vi "PI Terminal.vi"() -> ()   [LabVIEW 2014, in "PiFOC.lvlib"]
doc: "HELP for Terminal.vi\n\nThe terminal VI is a stand-alone application. It first asks the user to specify the full configuration (number of controlled systems, RS-232, GPIB, TCP-IP or DLL communication, communications parameters), then it establishes a connection with a selected system. This will work for all PI devices which support the PI General Command Set, or at least follow the same syntax rules and support the *IDN? and ERR? commands.\n\nAfter starting the VI, the interface parameters of the systems with which to communicate must be selected. For this reason, \"PITerminal.vi\" calls \"PI Ask for Communication Parameters.vi\". Select here the number of connected PI systems that you want to communicate with. For each system, select the appropriate interface parameters. \n\nC-702: Interface = RS232 or TCP/IP, RS232: Input and output HW handshake must be TRUE. Syntax: GCS 1.0; Term char = LF.\n\nC-843: Interface = DLL, DLL for Device = C-843, DLL Interface = Board, Parameter = Board number (1 for first C-843 board). Syntax: GCS 1.0; Term char = LF.\n\nC-843.PM: Interface = DLL, DLL for Device = C-843.PM, DLL Interface = Board, Parameter = Board number (1 for first C-843 board). Syntax: GCS 1.0; Term char = LF.\n\nC-844: Interface = DLL, DLL for Device = C-844, DLL Interface = RS232 or GPIB, Parameter = empty string, RS232 baud rate = 9600. Syntax: GCS 1.0; Term char = LF.\n\nC-865: Interface = DLL, DLL for Device = C-865, DLL Interface = RS232, Parameter = empty string, RS232 baud rate = set as appropriate. Syntax: GCS 1.0; Term char = LF.\n\nC-866: Interface = DLL, DLL for Device = C-866, DLL Interface = RS232 or USB, RS232: Parameter = empty string, RS232 baud rate = set as appropriate, USB: Parameter = Serial no. of system to connect to, Syntax: GCS 1.0; Term char = LF.\n\nC-867: Single Device: Interface = RS232 or DLL, RS232: Input and output HW handshake must be FALSE. DLL (USB): DLL for Device = C-867, DLL Interface = USB, Parameter = Serial no. of system to connect to. DaisyChain: Interface = DLL, DLL for Device = C-867, DLL Interface = RS232_DC, Parameter = Number of device in chain, Register DC: FALSE. Syntax: GCS 2.0; Term char = LF.\n\nC-880, C-848: Interface = RS232 or GPIB, RS232: Input and output HW handshake must be TRUE. Syntax: GCS 1.0; Term char = LF.\n\nC-880K005: Interface = RS232, Input and output HW handshake must be FALSE. Syntax: GCS 1.0; Term char = LF.\n\nC-884: Interface = RS232, TCP/IP or DLL, RS232: Input and output HW handshake must be FALSE. DLL (USB): DLL for Device = PI_GCS2_DLL, DLL Interface = USB, Parameter = Serial no. of system to connect to. Syntax: GCS 2.0; Term char = LF.\n\nE-516: Interface = RS232 or GPIB, RS232: Input and output HW handshake must be TRUE. Syntax: GCS 1.0; Term char = LF.\n\nE-517: Interface = RS232, GPIB, TCP/IP or DLL, RS232: Input and output HW handshake must be TRUE, DLL (USB): DLL for Device = E-517, DLL Interface = USB, Parameter = Serial no. of system to connect to. Syntax: GCS 2.0; Term char = LF.\n\nE-709: Interface = RS232 or DLL, RS232: Input and output HW handshake must be TRUE. DLL (USB): DLL for Device = E-709, DLL Interface = USB, Parameter = Serial no. of system to connect to. Syntax: GCS 2.0; Term char = LF.\n\nE-710: Interface = DLL, DLL for Device = E-710, DLL Interface = RS232 or GPIB, Parameter = empty string. Syntax: GCS 1.0; Term char = LF.\n\nE-712: Interface = RS232, TCP/IP or DLL, RS232: Input and output HW handshake must be TRUE. DLL: DLL for Device = E-712, DLL Interface = USB, Parameter = Serial no. of system to connect to. Syntax: GCS 2.0; Term char = LF.\n\nE-725: Interface = RS232, TCP/IP or DLL, RS232: Input and output HW handshake must be TRUE. DLL: DLL for Device = E-725, DLL Interface = USB, Parameter = Serial no. of system to connect to. Syntax: GCS 2.0; Term char = LF.\n\nE-753: Interface = RS232 or TCP/IP, RS232: Input and output HW handshake must be TRUE. Syntax: GCS 2.0; Term char = LF.\n\nE-755: Single Device: Interface = RS232, Input and output HW handshake must be TRUE. DaisyChain: Interface = DLL, DLL for Device = E-755, DLL Interface = RS232_DC, Parameter = Number of device in chain (first device: 1). Syntax: GCS 2.0; Term char = LF.\n\nE-761: Interface = DLL, DLL for Device = E-761, DLL Interface = Board, Parameter = Board number (1 for first E-761 board). Syntax: GCS 1.0; Term char = LF.\n\nE-816: Interface = RS232 or DLL, RS232: Input and output HW handshake must be TRUE. DLL (USB): DLL for Device = E-816, DLL Interface = USB, Parameter = Serial no. of system to connect to. Syntax: GCS 1.0; Term char = LF. \n\nE-861: Single Device: Interface = RS232 or DLL, RS232: Input and output HW handshake must be FALSE. DLL (USB): DLL for Device = E-861, DLL Interface = USB, Parameter = Serial no. of system to connect to. DaisyChain: Interface = DLL, DLL for Device = E-861, DLL Interface = RS232_DC, Parameter = Number of device in chain (first device: 1), Register DC: FALSE. Syntax: GCS 2.0; Term char = LF.\n\nE-870: Interface = DLL, DLL (USB): DLL for Device = PI_GCS2_DLL, DLL Interface = USB, Parameter = Serial no. of system to connect to.\n Syntax: GCS 2.0; Term char = LF.\n\nE-871: Single Device: Interface = RS232 or DLL, RS232: Input and output HW handshake must be FALSE. DLL (USB): DLL for Device = PI_GCS2_DLL, DLL Interface = USB, Parameter = Serial no. of system to connect to.\n DaisyChain: Interface = DLL, DLL for Device = PI_GCS2_DLL, DLL Interface = RS232_DC or USB_DC, Parameter = Number of device in chain, Register DC: FALSE. Syntax: GCS 2.0; Term char = LF.\n\nHydra, Pollux: Interface = DLL, DLL (TCP/IP and RS-232): DLL for Device = PI_HydraPollux_GCS2_DLL, DLL Interface = RS232 or TCP/IP, Syntax: GCS 2.0; Term char = LF.\n\nF-206, M-8X0: For GCS syntax version = GCS 1.0 (older firmware or compatibility mode, can be set with CSV.vi), Interface = RS232, GPIB (not available for C-887 controller) or TCP/IP., The error status will not be cleared by this VI. The first ERR? query will report a hidden error with error code 1, which will be cleared during system initialization (INI). RS232: Input and output handshake settings must be FALSE. Syntax: GCS 1.0; Term char = LF.\n For GCS syntax version = GCS 2.0 (C-887 Controller), Interface = RS232 or TCP/IP. RS232: Input and output handshake settings must be FALSE. Syntax: GCS 2.0; Term char = LF.\n\nMercury™: Interface = DLL, DLL for Device = Mercury™, DLL Interface = RS232 (even if using USB), Parameter = empty string, RS232 baud rate = same as set on controller hardware. Syntax: GCS 1.0; Term char = LF.\n\nGCS_Mercury: Single Device: Interface = RS232 or DLL, RS232: Input and output HW handshake must be FALSE. DLL (USB): DLL for Device = PI_GCS2_DLL, DLL Interface = USB, Parameter = Serial no. of system to connect to.\n DaisyChain: Interface = DLL, DLL for Device = PI_GCS2_DLL, DLL Interface = RS232_DC, Parameter = Number of device in chain, Register DC: FALSE. Syntax: GCS 2.0; Term char = LF.\n\nIf the chosen timeout value is greater than 1000 ms, it will automatically be set to 1000 ms for a fluid program operation. \n\nIn the upper window (\"Send\") the user can enter commands which will be transmitted to the chosen device one line at a time when the ENTER key is pressed. \nAll controller responses are displayed in the Receive response window, which can be cleared by pressing the Clear Receive Window button or F2. \n\nThe view style of the Receive window can be changed to Show all characters or Hex View using the menu ring above the Receive window.\n\nExit or F10 will terminate the terminal application. \n\nTo send the last command again, just press the ENTER key again. The next line will then show the following entry: \"(Send: cmd)\" with cmd being the command from the line before, which was resent.\n\nWhen the terminal application has just been started, pressing ENTER without entering a command will send \"*IDN?\" to the chosen system. \n\nNew commands can only be inserted into the last line of the Send window. The user can scroll through the history of the Send window using the scroll bar or the cursor up/down keys, but cannot change the history or resend commands by pressing ENTER unless in the last line. Pressing ENTER will always resend the last command, no matter where the cursor is positioned. Selecting text and using copy and paste (Ctrl+C, Ctrl+V) works for single lines, if only the contents of one single line (the command text) is selected and copied, not the full line (including the LineFeed) or multiple lines.\n\nMany of PI's General Command Set compatible devices support single-byte commands. For example, the user can stop a fast scan of a C-880 or F-206 by sending an ASCII 24 (decimal). To enter this command into the Send window simply type a \"#\" followed by the decimal value of the byte to be sent, e.g. enter \"#24\" and presses ENTER to stop a fast scan. An entry \"(Send: *)\" will be added to the original command with * being the corresponding ASCII character of the single byte sent. \n\nPressing F1 or the Help button will pop up a help window. To return to the terminal application, press Esc. If Send ERR? on Exit? is TRUE, an \"ERR?\" query is sent to the device when Exit is pressed to prevent the controller from keeping an error condition produced during the use of the terminal application."
uses:
  PiFOC.lvlib
  Low Level/Communication.llb/Termination character.ctl
  Low Level/Communication.llb/Available DLLs.ctl
panel:
  out "Help string":string="\nHELP for PI Terminal.vi\nPress Esc to return to the terminal application.\n\nThis terminal application works for all PI devices which support the PI General Command Set or at least follow the syntax rules of this command structure and support the commands *IDN? and ERR?.\n\nIn the upper window (\"Send\") the user can enter commands which will be transmitted to the chosen device one line at a time when the ENTER key is pressed. All controller responses are displayed in the Receive response window, which can be cleared by pressing the Clear Receive Window button or F2. The view style of the Receive window can be changed to Show all characters or Hex View using the menu ring above the Receive window.\n\nExit or F10 will terminate the terminal application. \n\nTo send the last command again, just press the ENTER key again. The next line will then show the following entry: \"(Send: cmd)\" with cmd being the command from the line before, which was resent.\nWhen the terminal application has just been started, pressing ENTER without entering a command will send \"*IDN?\" to the chosen system.\n\nNew commands can only be inserted into the last line of the Send window. The user can scroll through the history of the Send window using the scroll bar or the cursor up/down keys, but cannot change the history or resend commands by pressing ENTER unless in the last line. Pressing ENTER will always resend the last command, no matter where the cursor is positioned. Selecting text and using copy and paste (Ctrl+C, Ctrl+V) works for single lines, if only the contents of one single line (the command text) is selected and copied, not the full line (including the LineFeed) or multiple lines.\n\nMany of PI's General Command Set compatible devices support single-byte commands. For example, the user can stop a fast scan of a C-880 or F-206 by sending an ASCII 24 (decimal). To enter this command into the Send window simply type a \"#\" followed by the decimal value of the byte to be sent, e.g. enter \"#24\" and presses ENTER to stop a fast scan. An entry \"(Send: *)\" will be added to the original command with * being the corresponding ASCII character of the single byte sent. \n\nIf Send ERR? on Exit? is TRUE, a \"ERR?\" query is sent to the device when Exit is pressed to prevent the controller from keeping an error condition produced during the use of the terminal application.\n\nC-702: \tInterface = RS232 or TCP/IP, RS232: Input and output HW handshake \tmust \tbe TRUE. Syntax: GCS 1.0; Term char = LF.\n\nC-843: \tInterface = DLL, DLL for Device = C-843, DLL Interface = Board, \tParameter = Board number (1 for first C-843 board). Syntax: GCS 1.0; \tTerm char = LF.\n\nC-843.PM: \tInterface = DLL, DLL for Device = C-843.PM, DLL Interface = Board, \tParameter = Board number (1 for first C-843 board). Syntax: GCS 1.0; \tTerm char = LF.\n\nC-865: \tInterface = DLL, DLL for Device = C-865, DLL Interface = RS232, \tParameter = empty string, RS232 baud rate = set as appropriate. Syntax: \tGCS 1.0; Term char = LF.\n\nC-866: \tInterface = DLL, DLL for Device = C-866, DLL Interface = RS232 or USB, \tRS232: Parameter = empty string, RS232 baud rate = set as appropriate, \tUSB: Parameter = Serial no. of system to connect to, \n\tSyntax: GCS 1.0; Term char = LF.\n\nC-867: \tSingle Device: Interface = RS232 or DLL, RS232: Input and output HW \thandshake must be FALSE. DLL (USB): DLL for Device = C-867, DLL \tInterface = USB, Parameter = Serial no. of system to connect to.\nDaisyChain: Interface = DLL, DLL for Device = C-867, DLL Interface = \tRS232_DC, Parameter = Number of device in chain, \tRegister DC: \tFALSE. Syntax: GCS 2.0; Term char = LF.\n\nC-880, C-848: \tInterface = RS232 or GPIB, RS232: Input and output HW handshake must \tbe TRUE. Syntax: GCS 1.0; Term char = LF.\n\nC-880K005: \tInterface = RS232, Input and output HW handshake must be FALSE. \tSyntax: GCS 1.0; Term char = LF.\n\nC-884: \tInterface = RS232, TCP/IP or DLL, RS232: Input and output HW handshake must be FALSE. DLL (USB): DLL for Device = PI_GCS2_DLL, DLL Interface = USB, Parameter = Serial no. of system to connect to. Syntax: GCS 2.0; Term char = LF.\n\nE-516: \tInterface = RS232 or GPIB, RS232: Input and output HW handshake must \tbe TRUE. Syntax: GCS 1.0; Term char = LF.\n\nE-517: \tInterface = RS232, GPIB, TCP/IP or DLL, RS232: Input and output HW \thandshake must be TRUE, DLL (USB): DLL for Device = E-517, DLL \tInterface = USB, Parameter = Serial no. of system to connect to. \nSyntax: GCS 2.0; Term char = LF.\n\nE-709: \tInterface = RS232 or DLL, RS232: Input and output HW handshake \tmust be TRUE. DLL (USB): DLL for Device = E-709, DLL Interface = USB, \tParameter = Serial no. of system to connect to. Syntax: GCS 2.0; Term \tchar = LF.\n\nE-710:\tInterface = DLL, DLL for Device = E-710, DLL Interface = RS232 or GPIB, \tParameter = empty string. Syntax: GCS 1.0; Term char = LF.\n\nE-712: \tInterface = RS232, TCP/IP or DLL, RS232: Input and output HW \thandshake must be TRUE. DLL: DLL for Device = E-712, DLL Interface = \tUSB, \tParameter = Serial no. of system to connect to. \n\tSyntax: GCS 2.0; Term char = LF.\n\nE-725: \tInterface = RS232, TCP/IP or DLL, RS232: Input and output HW \thandshake must be TRUE. DLL: DLL for Device = E-725, DLL Interface = \tUSB, \tParameter = Serial no. of system to connect to. \nSyntax: GCS 2.0; Term char = LF.\n\nE-753: \tInterface = RS232 or TCP/IP, RS232: Input and output HW handshake \tmust \tbe TRUE. Syntax: GCS 2.0; Term char = LF.\n\nE-755:\tSingle Device: Interface = RS232, Input and output HW handshake must \tbe TRUE. DaisyChain: Interface = DLL, DLL for Device = E-755, DLL \tInterface = RS232_DC, Parameter = Number of device in chain (first \tdevice: 1). Syntax: GCS 2.0; Term char = LF.\n\nE-761:\tInterface = DLL, DLL for Device = E-761, DLL Interface = Board, \tParameter = Board number (1 for first E-761 board). Syntax: GCS 1.0; \tTerm char = LF.\n\nE-816: \tInterface = RS232 or DLL, RS232: Input and output HW handshake must \tbe TRUE. DLL (USB): DLL for Device = E-816, DLL Interface = USB, \tParameter = Serial no. of system to connect to. Syntax: GCS 1.0; Term \tchar = LF. \n\nE-861: \tSingle Device: Interface = RS232 or DLL, RS232: Input and output HW \thandshake must be FALSE. DLL (USB): DLL for Device = E-861, DLL \tInterface = USB, Parameter = Serial no. of system to connect to.\nDaisyChain: Interface = DLL, DLL for Device = E-861, DLL Interface = \tRS232_DC or USB_DC, Parameter = Number of device in chain (first device: 1), \tRegister DC: FALSE. Syntax: GCS 2.0; Term char = LF.\n\nE-870: \tInterface = DLL, DLL (USB): DLL for Device = PI_GCS2_DLL, DLL \tInterface = USB, Parameter = Serial no. of system to connect to.\n\tSyntax: GCS 2.0; Term char = LF.\n\nE-871: Single Device: Interface = RS232 or DLL, RS232: Input and output HW \thandshake must be FALSE. DLL (USB): DLL for Device = \tPI_GCS2_DLL, DLL Interface = USB, Parameter = Serial no. of system to \tconnect to.\n\tDaisyChain: Interface = DLL, DLL for Device = PI_GCS2_DLL, DLL \tInterface = RS232_DC or USB_DC, Parameter = Number of device in \tchain, Register DC: FALSE. Syntax: GCS 2.0; Term char = LF.\n\nHydra, Pollux: \tInterface = DLL, DLL (TCP/IP and RS-232): DLL for Device = \t\t\t\t\tPI_HydraPollux_GCS2_DLL, DLL Interface = RS232 or TCP/IP, Syntax: \t\t\tGCS 2.0; Term char = LF.\n\nF-206, M-8X0: \tFor GCS syntax version = GCS 1.0 (older firmware or compatibility mode, \tcan be set with CSV.vi), Interface = RS232, GPIB (not available for C-887 \tcontroller) or TCP/IP., The error status will not be cleared by this VI. The \tfirst ERR? query will report a hidden error with error code 1, which will be \tcleared during system initialization (INI). RS232: Input and output \thandshake settings must be FALSE. Syntax: GCS 1.0; Term char = \tLF.\n\tFor GCS syntax version = GCS 2.0 (C-887 Controller), Interface = RS232 \tor TCP/IP. RS232: Input and output handshake settings must be FALSE. \tSyntax: GCS 2.0; Term char = LF.\n\nMercury™: \tInterface = DLL, DLL for Device = Mercury™, DLL Interface = RS232 \t(even if using USB), Parameter = empty string, RS232 baud rate = same \tas set on controller hardware, Syntax: GCS 1.0; Term char = LF.\n\nGCS_Mercury: \tSingle Device: Interface = RS232 or DLL, RS232: Input and output HW \thandshake must be FALSE. DLL (USB): DLL for Device = PI_GCS2_DLL, \tDLL Interface = USB, Parameter = Serial no. of system to connect to. \tDaisyChain: Interface = DLL, DLL for Device = PI_GCS2_DLL, DLL \tInterface = RS232_DC or USB_DaisyChain, Parameter = Number of device in chain, \tRegister DC: \tFALSE. Syntax: GCS 2.0; Term char = LF.\n"
  in  "HowTo":string="Start application and choose interface parameters in next window."
  out "TCP/IP Config. System":T1={"Host address/name"="Z-A521-2.pi.ws", "Port"=3000, "Board"=0, "Timeout"=5000}
  in  "ERR? on exit?":bool=TRUE
  out "error out":T2
  out "GPIB Configuration system":T3={"bus"=0, "address"=4, "mode"=0, "Timeout"=1000}
  in  "Hide help":bool
  in  "Show help":bool
  in  "View style":u16(ring) items=["Normal view", "Show all characters", "Hex View"]
  out "error":bool
  in  "Send":bool
  in  "Clear":bool
  in  "Exit":bool
  out "Receive":string
  in  "System No.":i32=1 min=1 step=1
  out "Interface":u16(ring) items=["RS232", "GPIB", "DLL", "TCP/IP"]
  out "System ind.":i32=1
  out "System":i32=1
  out "RS232 Config. System":T4={"RS232 Portnumber"=0, "Timeout"=1000, "Baudrate"=57600, "Handshake"=0} {"Handshake" items=["None", "HW", "XON/XOFF"]; "RS232 Portnumber" items=["COM1", "COM2", "COM3", "COM4", "COM5", "COM6", "COM7", "COM8", "COM9", "COM10", "COM11", "COM12", "COM13", "COM14", "COM15", "COM16", "COM17", "COM18", "COM19", "COM20", "COM21", "COM22", "COM23", "COM24", "COM25", "COM26", "COM27", "COM28", "COM29", "COM30"]}
  in  "Send":string="*IDN?\n"
  out "Term.char":T5
  out "DLL for Device":T6 items=["C-843", "C-844", "E-710", "C-843.PM", "C-865", "E-761", "Mercury", "E-755", "E-753", "C-866", "E-712", "E-725", "E-861", "C-867", "E-517", "E-816", "E-709", "PI_GCS2_DLL", "HydraPollux"]
  # "Terminal"
  # "If chosen timeout value is > 1000 ms, \nit will be set to 300 ms."
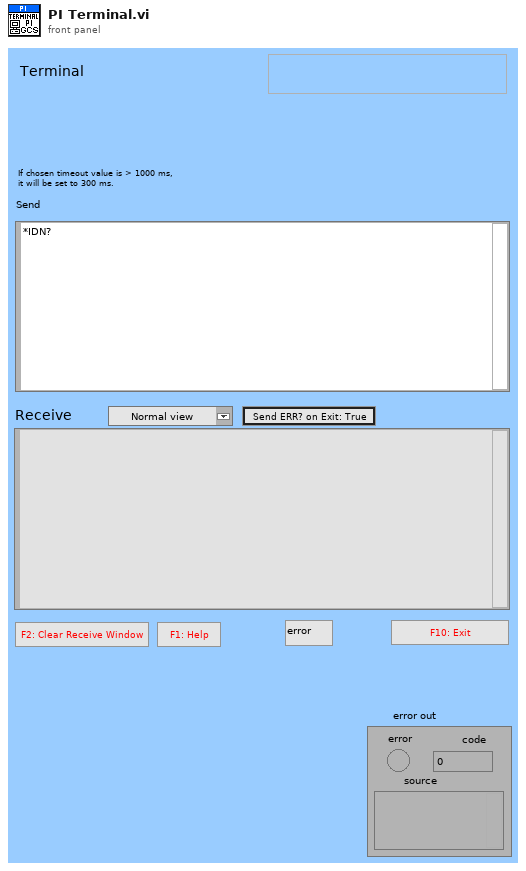
[diagram p1: front panel]
types:
  T1 = cluster{"Host address/name":string, "Port":i32, "Board":i32, "Timeout":i32}
  T2 = cluster{"error":bool, "code":i32, "source":string}
  T3 = cluster{"bus":i16, "address":i16, "mode":i16, "Timeout":i32}
  T4 = cluster{"RS232 Portnumber":i32, "Timeout":i32, "Baudrate":u32, "Handshake":u16}
  T5 = typedef "PiFOC.lvlib/Termination character.ctl" = enum16{"LF", "CR", "LFCR", "CRLF"}
  T6 = typedef "PiFOC.lvlib/Available DLLs.ctl" = u16
  T7 = cluster{"data bits":u16, "stop bits":enum16{"1 bit", "1.5 bits", "2 bits"}, "parity":enum16{"no parity", "odd parity", "even parity", "mark parity", "space parity"}}
  T8 = cluster{"Host address/name":string, "Port":i32, "Board":i32}[]
  T9 = cluster{"input XON/XOFF":bool, "input HW Handshake":bool, "input alt HW HShk":bool, "output XON/XOFF":bool, "output HW Handshake":bool, "output alt HW HShk":bool, "XOFF byte ":u8, "XON byte":u8, "parity error byte":u16}[]
  T10 = typedef "PiFOC.lvlib/Available interfaces.ctl" = u16
  T11 = cluster{"RS232 Portnumber":u16, "Timeout":u32, "RS232 baud rate":u32, "Interface":T10, "GPIB Bus":i16, "GPIB address":i16, "GPIB Mode":i16}[]
  T12 = typedef "PiFOC.lvlib/Available DLL interfaces.ctl" = u16
  T13 = cluster{"DLL for Device":T6, "DLL Interface":T12, "Parameter":string}[]
  T14 = cluster{"RS232 Portnumber":u16, "Timeout":u32, "RS232 baud rate":u32, "Interface":T10, "GPIB Bus":i16, "GPIB address":i16, "GPIB Mode":i16}
  T15 = cluster{"Portnumber":u32, "Timeout":i32, "Baudrate":u32, "Handshake":u16}
  T16 = cluster{"data bits":u16, "stop bits":enum16{"1 bit", "1.5 bits", "2 bits"}, "parity":enum16{"no parity", "odd parity", "even parity", "mark parity", "space parity"}}[]
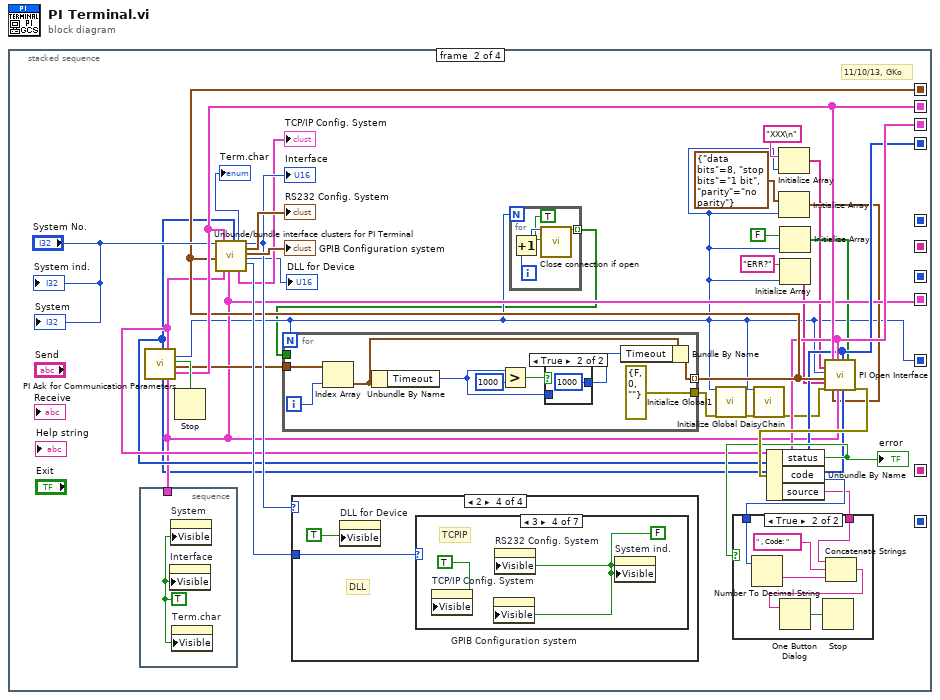
[diagram p0: block diagram]
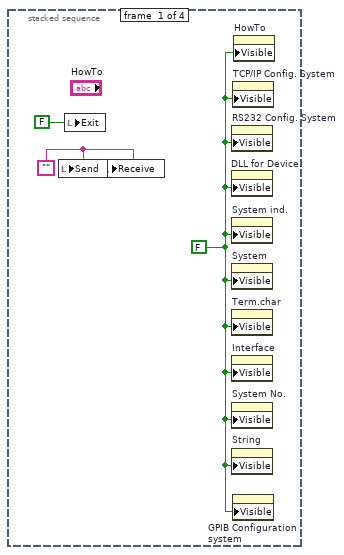
[diagram p2: hidden frame]
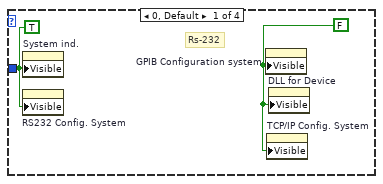
[diagram p3: hidden frame]
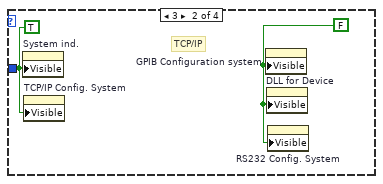
[diagram p4: hidden frame]
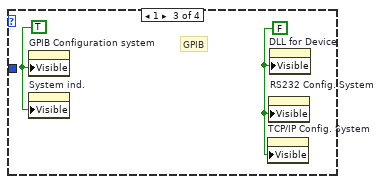
[diagram p5: hidden frame]
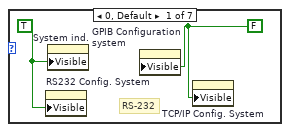
[diagram p6: hidden frame]
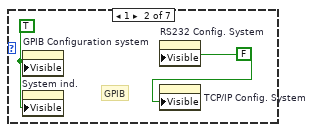
[diagram p7: hidden frame]
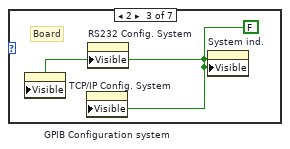
[diagram p8: hidden frame]
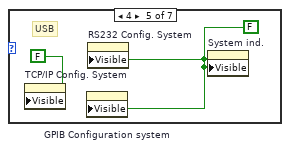
[diagram p9: hidden frame]
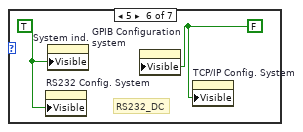
[diagram p10: hidden frame]
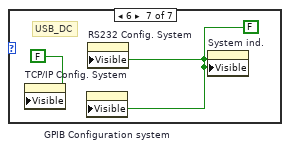
[diagram p11: hidden frame]
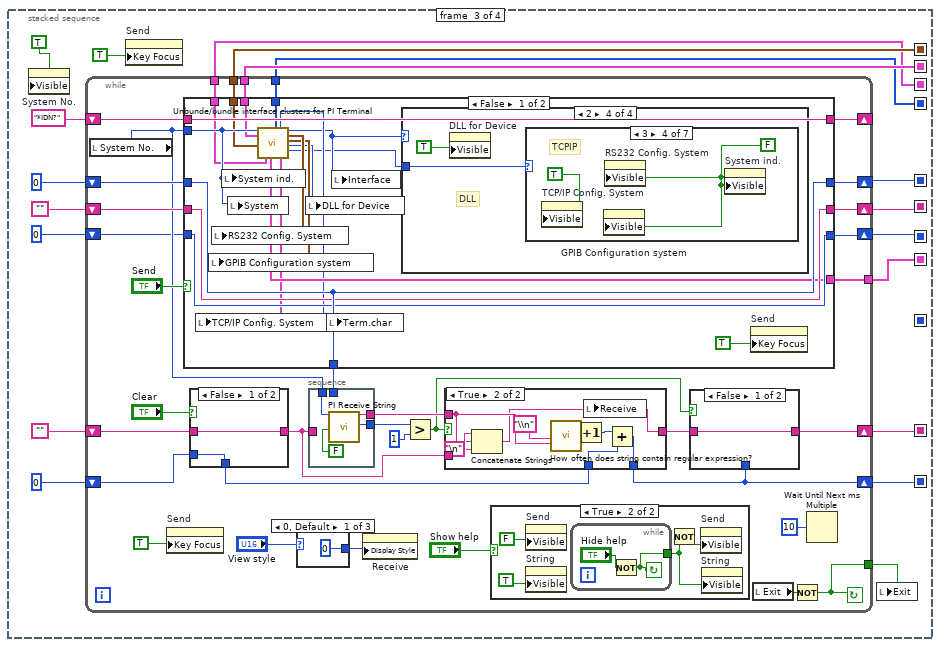
[diagram p14: hidden frame]
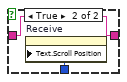
[diagram p16: hidden frame]
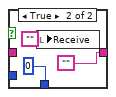
[diagram p17: hidden frame]
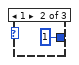
[diagram p19: hidden frame]
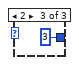
[diagram p20: hidden frame]
diagram:
  n1 = stacked-sequence {
    seq-local: [_ w24 _ _] -> [_ _ w97 _]
    seq-local: [_ w32 _ _] -> [_ _ w96 _]
    seq-local: [_ w19 _ _] -> [_ _ w87 _]
    seq-local: [_ _ w86 _] -> [_ _ _ w246]
    seq-local: [_ _ w85 _] -> [_ _ _ w245]
    seq-local: [_ _ w84 _] -> [_ _ _ w247]
    seq-local: [_ _ w83 _] -> [_ _ _ w248]
    seq-local: [_ _ w82 _] -> [_ _ _ w249]
    seq-local: [_ w21 _ _] -> [_ _ w81 _]
    seq-local: [_ w20 _ _] -> [_ _ w80 _]
    seq-local: [_ w7 _ _] -> [_ _ _ w243]
    frame #0 {
      w1 = FALSE ("Visible")
      w3 = ""
      n2 = local write "Send"(w3) -> ()
      n3 = local write "Exit"(FALSE ("error")) -> ()
      n4 = local write "Receive"(w3) -> ()
      n5 = property on="RS232 Config. System" class="Clust (strict)"("Visible"=w1) -> ()  [unwired: 2 in, 2 out]
      n6 = property on="DLL for Device" class="Ring (strict)"("Visible"=w1) -> ()  [unwired: 2 in, 2 out]
      n7 = property on="System ind." class="DigNum (strict)"("Visible"=w1) -> ()  [unwired: 2 in, 2 out]
      n8 = property on="System" class="DigNum (strict)"("Visible"=w1) -> ()  [unwired: 2 in, 2 out]
      n9 = property on="Term.char" class="Enum (strict)"("Visible"=w1) -> ()  [unwired: 2 in, 2 out]
      n10 = property on="Interface" class="Ring (strict)"("Visible"=w1) -> ()  [unwired: 2 in, 2 out]
      n11 = property on="System No." class="DigNum (strict)"("Visible"=w1) -> ()  [unwired: 2 in, 2 out]
      n12 = property on="String" class="Str"("Visible"=w1) -> ()  [unwired: 2 in, 2 out]
      n13 = property on="TCP/IP Config. System" class="Clust (strict)"("Visible"=w1) -> ()  [unwired: 2 in, 2 out]
      n14 = property on="GPIB Configuration system" class="Clust (strict)"("Visible"=w1) -> ()  [unwired: 2 in, 2 out]
      n15 = property on="HowTo" class="Str"("Visible"=w1) -> ()  [unwired: 2 in, 2 out]
    }
    frame #1 {
      # "11/10/13, GKo"
      n16 = call "PI Ask for Communication Parameters.vi"() -> ("Termination character out"=w20:T5[], "Syntax out"=w18:enum16{"GCS 1.0", "GCS 2.0"}[], "TCP/IP Configuration out"=w21:T8, "Flow control out"=w19:T9, "How many\nsystems? out"=w7:i32, "Abort out"=w35:bool, "Interface configuration out"=w25:T11, "DLL Interface\nconfiguration out"=w32:T13)  [unwired: 12 out]
      n17 = stacked-sequence {
        tunnel: w19 -> [_]
        frame #0 {
          w41 = TRUE ("Visible")
          n18 = property on="Interface" class="Ring (strict)"("Visible"=w41) -> ()  [unwired: 2 in, 2 out]
          n19 = property on="System" class="DigNum (strict)"("Visible"=w41) -> ()  [unwired: 2 in, 2 out]
          n20 = property on="Term.char" class="Enum (strict)"("Visible"=w41) -> ()  [unwired: 2 in, 2 out]
        }
      }
      n21 = Stop(stop? (T)=w35) -> ()
      n22 = for {
        N: w7 -> [_]
        tunnel: [w37] -> w6 mode=indexing
        i -> [w40]
        n23 = Increment(x=w40) -> (x+1=w39:i32)
        n24 = call "Close connection if open.vi"("System no."=w39, "Close DaisyChain"=TRUE) -> ("Was connected?"=w37:bool)  [unwired: 1 in, 16 out]
      }
      n25 = for {
        N: w7 -> [_]
        tunnel: w25 -> [w76]
        tunnel: [w75] -> w24 mode=indexing
        tunnel: w6 -> [_]
        tunnel: [errorcluster {"status"=FALSE, "code"=0, "source"=""} ("error in")] -> w5
        i -> [w77]
        n26 = Index Array(array=w76, index=w77) -> (element=w72:T14)
        n27 = Unbundle By Name(w72) -> ("Timeout"=w71:u32)
        n28 = Greater?(x=w71, y=u32 1000) -> (0:w70:bool)
        n29 = case shown="True" w70 {
          tunnel: [w78 1000] -> w73
          tunnel: w71 -> [w78 _]
          frame False {
          }
          frame True {
          }
        }
        n30 = Bundle By Name(cluster=w72, "Timeout"=w73) -> (w75:T14)
      }
      n31 = call "Unbunde/bundle interface clusters for PI Terminal.vi"("System No."="System No.", "Interface configuration"=w24, "DLL Interface\nconfiguration"=w32, "TCP/IP Configuration"=w21, "Flow control"=w19, "Termination character"=w20) -> ("Term.char"=→"Term.char":T5, "TCP/IP Config. System"=→"TCP/IP Config. System":T1, "Interface"=w28:T10, "RS232 configuration system"=→"RS232 Config. System":T15, "GPIB configuration system"=→"GPIB Configuration system":T3, "DLL for Device"=→"DLL for Device":T6, "DLL interface"=w27:T12)  [unwired: 7 out]
      "Interface" <- w28
      n32 = case shown="2" w28 {
        tunnel: w27 -> [_ _ _ w49]
        frame 0, Default {
          w42 = FALSE ("Write Attribute")
          w43 = TRUE ("Write Attribute")
          # "Rs-232"
          n33 = property on="System ind." class="DigNum (strict)"("Visible"=w43) -> ()  [unwired: 2 in, 2 out]
          n34 = property on="RS232 Config. System" class="Clust (strict)"("Visible"=w43) -> ()  [unwired: 2 in, 2 out]
          n35 = property on="GPIB Configuration system" class="Clust (strict)"("Visible"=w42) -> ()  [unwired: 2 in, 2 out]
          n36 = property on="TCP/IP Config. System" class="Clust (strict)"("Visible"=w42) -> ()  [unwired: 2 in, 2 out]
          n37 = property on="DLL for Device" class="Ring (strict)"("Visible"=w42) -> ()  [unwired: 2 in, 2 out]
        }
        frame 3 {
          w44 = FALSE ("Write Attribute")
          w45 = TRUE ("Write Attribute")
          # "TCP/IP"
          n38 = property on="System ind." class="DigNum (strict)"("Visible"=w45) -> ()  [unwired: 2 in, 2 out]
          n39 = property on="TCP/IP Config. System" class="Clust (strict)"("Visible"=w45) -> ()  [unwired: 2 in, 2 out]
          n40 = property on="GPIB Configuration system" class="Clust (strict)"("Visible"=w44) -> ()  [unwired: 2 in, 2 out]
          n41 = property on="DLL for Device" class="Ring (strict)"("Visible"=w44) -> ()  [unwired: 2 in, 2 out]
          n42 = property on="RS232 Config. System" class="Clust (strict)"("Visible"=w44) -> ()  [unwired: 2 in, 2 out]
        }
        frame 1 {
          w47 = TRUE ("Write Attribute")
          w46 = FALSE ("Write Attribute")
          # "GPIB"
          n43 = property on="GPIB Configuration system" class="Clust (strict)"("Visible"=w47) -> ()  [unwired: 2 in, 2 out]
          n44 = property on="System ind." class="DigNum (strict)"("Visible"=w47) -> ()  [unwired: 2 in, 2 out]
          n45 = property on="TCP/IP Config. System" class="Clust (strict)"("Visible"=w46) -> ()  [unwired: 2 in, 2 out]
          n46 = property on="RS232 Config. System" class="Clust (strict)"("Visible"=w46) -> ()  [unwired: 2 in, 2 out]
          n47 = property on="DLL for Device" class="Ring (strict)"("Visible"=w46) -> ()  [unwired: 2 in, 2 out]
        }
        frame 2 {
          # "DLL"
          n48 = property on="DLL for Device" class="Ring (strict)"("Visible"=TRUE ("Write Attribute")) -> ()  [unwired: 2 in, 2 out]
          n49 = case shown="3" w49 {
            frame 0, Default {
              w50 = FALSE ("Write Attribute")
              w51 = TRUE ("Write Attribute")
              # "RS-232"
              n50 = property on="RS232 Config. System" class="Clust (strict)"("Visible"=w51) -> ()  [unwired: 2 in, 2 out]
              n51 = property on="System ind." class="DigNum (strict)"("Visible"=w51) -> ()  [unwired: 2 in, 2 out]
              n52 = property on="GPIB Configuration system" class="Clust (strict)"("Visible"=w50) -> ()  [unwired: 2 in, 2 out]
              n53 = property on="TCP/IP Config. System" class="Clust (strict)"("Visible"=w50) -> ()  [unwired: 2 in, 2 out]
            }
            frame 1 {
              w53 = TRUE ("Write Attribute")
              w52 = FALSE ("Write Attribute")
              # "GPIB"
              n54 = property on="GPIB Configuration system" class="Clust (strict)"("Visible"=w53) -> ()  [unwired: 2 in, 2 out]
              n55 = property on="System ind." class="DigNum (strict)"("Visible"=w53) -> ()  [unwired: 2 in, 2 out]
              n56 = property on="RS232 Config. System" class="Clust (strict)"("Visible"=w52) -> ()  [unwired: 2 in, 2 out]
              n57 = property on="TCP/IP Config. System" class="Clust (strict)"("Visible"=w52) -> ()  [unwired: 2 in, 2 out]
            }
            frame 2 {
              w54 = FALSE ("Write Attribute")
              # "Board"
              n58 = property on="TCP/IP Config. System" class="Clust (strict)"("Visible"=w54) -> ()  [unwired: 2 in, 2 out]
              n59 = property on="GPIB Configuration system" class="Clust (strict)"("Visible"=w54) -> ()  [unwired: 2 in, 2 out]
              n60 = property on="RS232 Config. System" class="Clust (strict)"("Visible"=w54) -> ()  [unwired: 2 in, 2 out]
              n61 = property on="System ind." class="DigNum (strict)"("Visible"=w54) -> ()  [unwired: 2 in, 2 out]
            }
            frame 3 {
              w56 = FALSE ("Write Attribute")
              # "TCPIP"
              n62 = property on="TCP/IP Config. System" class="Clust (strict)"("Visible"=TRUE) -> ()  [unwired: 2 in, 2 out]
              n63 = property on="GPIB Configuration system" class="Clust (strict)"("Visible"=w56) -> ()  [unwired: 2 in, 2 out]
              n64 = property on="RS232 Config. System" class="Clust (strict)"("Visible"=w56) -> ()  [unwired: 2 in, 2 out]
              n65 = property on="System ind." class="DigNum (strict)"("Visible"=w56) -> ()  [unwired: 2 in, 2 out]
            }
            frame 4 {
              w58 = FALSE ("Write Attribute")
              # "USB"
              n66 = property on="TCP/IP Config. System" class="Clust (strict)"("Visible"=FALSE) -> ()  [unwired: 2 in, 2 out]
              n67 = property on="GPIB Configuration system" class="Clust (strict)"("Visible"=w58) -> ()  [unwired: 2 in, 2 out]
              n68 = property on="RS232 Config. System" class="Clust (strict)"("Visible"=w58) -> ()  [unwired: 2 in, 2 out]
              n69 = property on="System ind." class="DigNum (strict)"("Visible"=w58) -> ()  [unwired: 2 in, 2 out]
            }
            frame 5 {
              w59 = FALSE ("Write Attribute")
              w60 = TRUE ("Write Attribute")
              # "RS232_DC"
              n70 = property on="RS232 Config. System" class="Clust (strict)"("Visible"=w60) -> ()  [unwired: 2 in, 2 out]
              n71 = property on="System ind." class="DigNum (strict)"("Visible"=w60) -> ()  [unwired: 2 in, 2 out]
              n72 = property on="GPIB Configuration system" class="Clust (strict)"("Visible"=w59) -> ()  [unwired: 2 in, 2 out]
              n73 = property on="TCP/IP Config. System" class="Clust (strict)"("Visible"=w59) -> ()  [unwired: 2 in, 2 out]
            }
            frame 6 {
              w62 = FALSE ("Write Attribute")
              # "USB_DC"
              n74 = property on="TCP/IP Config. System" class="Clust (strict)"("Visible"=FALSE) -> ()  [unwired: 2 in, 2 out]
              n75 = property on="GPIB Configuration system" class="Clust (strict)"("Visible"=w62) -> ()  [unwired: 2 in, 2 out]
              n76 = property on="RS232 Config. System" class="Clust (strict)"("Visible"=w62) -> ()  [unwired: 2 in, 2 out]
              n77 = property on="System ind." class="DigNum (strict)"("Visible"=w62) -> ()  [unwired: 2 in, 2 out]
            }
          }
        }
      }
      n78 = call "Initialize Global1.vi"("System no."=w7, "error in"=w5) -> ("error out"=w17:errorcluster)  [unwired: 17 out]
      n79 = call "Initialize Global DaisyChain.vi"("System no."=w7, "error in"=w17) -> ("error out"=w16:errorcluster)  [unwired: 17 out]
      n80 = Initialize Array("XXX\n", w7) -> (w9:string[])
      n81 = Initialize Array(T7 {"data bits"=8, "stop bits"=enum."1 bit", "parity"=enum."no parity"} ("Bit settings and parity"), w7) -> (w11:T16)
      n82 = Initialize Array(FALSE ("Register DC"), w7) -> (w15:bool[])
      n83 = Initialize Array("ERR?", w7) -> (w13:string[])
      n84 = call "PI Open Interface.vi"("Interface clear"=w9, "Number of systems"=w7, "Interface configuration"=w24, "Strings to send"=w13, "error in"=w16, "DLL Interface\nConfiguration"=w32, "Bit settings and parity"=w11, "TCP/IP\nConfiguration"=w21, "Flow control"=w19, "Termination character"=w20, "Syntax"=w18, "Register DC"=w15) -> ("error out"=w36:errorcluster)  [unwired: 7 out]
      n85 = Unbundle By Name(w36) -> ("status"=w26:bool, "code"=w34:i32, "source"=w33:string)
      "error" <- w26
      n86 = case shown="True" w26 {
        tunnel: w34 -> [_ w67]
        tunnel: w33 -> [_ w66]
        frame False {
        }
        frame True {
          n87 = Number To Decimal String(number=w67) -> (decimal integer string=w64:string)  [unwired: 1 out]
          n88 = Concatenate Strings(w66, " , Code: " ("Substring"), w64) -> (w63:string)
          n89 = One Button Dialog(message=w63) -> (true=w68:bool)  [unwired: 1 out]
          n90 = Stop(stop? (T)=w68) -> ()
        }
      }
      "System ind." <- "System No."
      "System" <- "System No."
    }
    frame #2 {
      n91 = property on="System No." class="DigNum (strict)"("Visible"=TRUE ("Write Attribute")) -> ()  [unwired: 2 in, 2 out]
      n92 = while {
        tunnel: w87 -> [w102]
        tunnel: [w103] -> w88
        shift-left: 0 -> [w116]
        shift-right: [w115] -> w84
        shift-left: 0 -> [w112]
        shift-right: [w106] -> w85
        shift-left: "" -> [w113]
        shift-right: [w107] -> w86
        shift-left: "" -> [w124]
        shift-right: [w123] -> w83
        shift-left: 0 -> [w128]
        shift-right: [w127] -> w82
        tunnel: w96 -> [w132]
        tunnel: w97 -> [w133]
        shift-left: "*IDN?" -> [w130]
        shift-right: [w129] -> _
        tunnel: w81 -> [w100]
        tunnel: w80 -> [w99]
        stop <- w103 continue-if-true
        n93 = local read "System No."() -> (w121:i32)
        n94 = property on="Send" class="Str"("Key Focus"=TRUE ("Write Attribute")) -> ()  [unwired: 2 in, 2 out]
        n95 = case shown="False" "Send" {
          tunnel: w121 -> [w178 w224]
          tunnel: w133 -> [w177 _]
          tunnel: w132 -> [w176 _]
          tunnel: w130 -> [w183 w222]
          tunnel: [w183 w219] -> w129
          tunnel: w128 -> [w182 w210]
          tunnel: [w182 w207] -> w127
          tunnel: w124 -> [w179 w218]
          tunnel: [w179 w214] -> w123
          tunnel: [w182 w207] -> w122
          tunnel: w116 -> [w180 w213]
          tunnel: [w180 w209] -> w115
          tunnel: w102 -> [w172 _]
          tunnel: w100 -> [w171 _]
          tunnel: w99 -> [w170 _]
          frame False {
            n96 = local write "System ind."(w178) -> ()
            n97 = local write "System"(w178) -> ()
            n98 = call "Unbunde/bundle interface clusters for PI Terminal.vi"("System No."=w178, "Interface configuration"=w177, "DLL Interface\nconfiguration"=w176, "TCP/IP Configuration"=w171, "Flow control"=w172, "Termination character"=w170) -> ("Term.char"=w168:T5, "TCP/IP Config. System"=w169:T1, "Interface"=w167:T10, "RS232 configuration system"=w175:T15, "GPIB configuration system"=w174:T3, "DLL for Device"=w173:T6, "DLL interface"=w166:T12)  [unwired: 7 out]
            n99 = local write "TCP/IP Config. System"(w169) -> ()
            n100 = local write "GPIB Configuration system"(w174) -> ()
            n101 = local write "RS232 Config. System"(w175) -> ()
            n102 = local write "DLL for Device"(w173) -> ()
            n103 = local write "Term.char"(w168) -> ()
            n104 = local write "Interface"(w167) -> ()
            n105 = case shown="2" w167 {
              tunnel: w166 -> [_ _ _ w191]
              frame 0, Default {
                w184 = FALSE ("Write Attribute")
                w185 = TRUE ("Write Attribute")
                # "Rs-232"
                n106 = property on="System ind." class="DigNum (strict)"("Visible"=w185) -> ()  [unwired: 2 in, 2 out]
                n107 = property on="RS232 Config. System" class="Clust (strict)"("Visible"=w185) -> ()  [unwired: 2 in, 2 out]
                n108 = property on="GPIB Configuration system" class="Clust (strict)"("Visible"=w184) -> ()  [unwired: 2 in, 2 out]
                n109 = property on="TCP/IP Config. System" class="Clust (strict)"("Visible"=w184) -> ()  [unwired: 2 in, 2 out]
                n110 = property on="DLL for Device" class="Ring (strict)"("Visible"=w184) -> ()  [unwired: 2 in, 2 out]
              }
              frame 3 {
                w186 = FALSE ("Write Attribute")
                w187 = TRUE ("Write Attribute")
                # "TCP/IP"
                n111 = property on="System ind." class="DigNum (strict)"("Visible"=w187) -> ()  [unwired: 2 in, 2 out]
                n112 = property on="TCP/IP Config. System" class="Clust (strict)"("Visible"=w187) -> ()  [unwired: 2 in, 2 out]
                n113 = property on="GPIB Configuration system" class="Clust (strict)"("Visible"=w186) -> ()  [unwired: 2 in, 2 out]
                n114 = property on="DLL for Device" class="Ring (strict)"("Visible"=w186) -> ()  [unwired: 2 in, 2 out]
                n115 = property on="RS232 Config. System" class="Clust (strict)"("Visible"=w186) -> ()  [unwired: 2 in, 2 out]
              }
              frame 1 {
                w189 = TRUE ("Write Attribute")
                w188 = FALSE ("Write Attribute")
                # "GPIB"
                n116 = property on="GPIB Configuration system" class="Clust (strict)"("Visible"=w189) -> ()  [unwired: 2 in, 2 out]
                n117 = property on="System ind." class="DigNum (strict)"("Visible"=w189) -> ()  [unwired: 2 in, 2 out]
                n118 = property on="TCP/IP Config. System" class="Clust (strict)"("Visible"=w188) -> ()  [unwired: 2 in, 2 out]
                n119 = property on="RS232 Config. System" class="Clust (strict)"("Visible"=w188) -> ()  [unwired: 2 in, 2 out]
                n120 = property on="DLL for Device" class="Ring (strict)"("Visible"=w188) -> ()  [unwired: 2 in, 2 out]
              }
              frame 2 {
                # "DLL"
                n121 = property on="DLL for Device" class="Ring (strict)"("Visible"=TRUE ("Write Attribute")) -> ()  [unwired: 2 in, 2 out]
                n122 = case shown="3" w191 {
                  frame 0, Default {
                    w192 = FALSE ("Write Attribute")
                    w193 = TRUE ("Write Attribute")
                    # "RS-232"
                    n123 = property on="RS232 Config. System" class="Clust (strict)"("Visible"=w193) -> ()  [unwired: 2 in, 2 out]
                    n124 = property on="System ind." class="DigNum (strict)"("Visible"=w193) -> ()  [unwired: 2 in, 2 out]
                    n125 = property on="GPIB Configuration system" class="Clust (strict)"("Visible"=w192) -> ()  [unwired: 2 in, 2 out]
                    n126 = property on="TCP/IP Config. System" class="Clust (strict)"("Visible"=w192) -> ()  [unwired: 2 in, 2 out]
                  }
                  frame 1 {
                    w195 = TRUE ("Write Attribute")
                    w194 = FALSE ("Write Attribute")
                    # "GPIB"
                    n127 = property on="GPIB Configuration system" class="Clust (strict)"("Visible"=w195) -> ()  [unwired: 2 in, 2 out]
                    n128 = property on="System ind." class="DigNum (strict)"("Visible"=w195) -> ()  [unwired: 2 in, 2 out]
                    n129 = property on="RS232 Config. System" class="Clust (strict)"("Visible"=w194) -> ()  [unwired: 2 in, 2 out]
                    n130 = property on="TCP/IP Config. System" class="Clust (strict)"("Visible"=w194) -> ()  [unwired: 2 in, 2 out]
                  }
                  frame 2 {
                    w196 = FALSE ("Write Attribute")
                    # "Board"
                    n131 = property on="TCP/IP Config. System" class="Clust (strict)"("Visible"=w196) -> ()  [unwired: 2 in, 2 out]
                    n132 = property on="GPIB Configuration system" class="Clust (strict)"("Visible"=w196) -> ()  [unwired: 2 in, 2 out]
                    n133 = property on="RS232 Config. System" class="Clust (strict)"("Visible"=w196) -> ()  [unwired: 2 in, 2 out]
                    n134 = property on="System ind." class="DigNum (strict)"("Visible"=w196) -> ()  [unwired: 2 in, 2 out]
                  }
                  frame 3 {
                    w198 = FALSE ("Write Attribute")
                    # "TCPIP"
                    n135 = property on="TCP/IP Config. System" class="Clust (strict)"("Visible"=TRUE) -> ()  [unwired: 2 in, 2 out]
                    n136 = property on="GPIB Configuration system" class="Clust (strict)"("Visible"=w198) -> ()  [unwired: 2 in, 2 out]
                    n137 = property on="RS232 Config. System" class="Clust (strict)"("Visible"=w198) -> ()  [unwired: 2 in, 2 out]
                    n138 = property on="System ind." class="DigNum (strict)"("Visible"=w198) -> ()  [unwired: 2 in, 2 out]
                  }
                  frame 4 {
                    w200 = FALSE ("Write Attribute")
                    # "USB"
                    n139 = property on="TCP/IP Config. System" class="Clust (strict)"("Visible"=FALSE) -> ()  [unwired: 2 in, 2 out]
                    n140 = property on="GPIB Configuration system" class="Clust (strict)"("Visible"=w200) -> ()  [unwired: 2 in, 2 out]
                    n141 = property on="RS232 Config. System" class="Clust (strict)"("Visible"=w200) -> ()  [unwired: 2 in, 2 out]
                    n142 = property on="System ind." class="DigNum (strict)"("Visible"=w200) -> ()  [unwired: 2 in, 2 out]
                  }
                  frame 5 {
                    w201 = FALSE ("Write Attribute")
                    w202 = TRUE ("Write Attribute")
                    # "RS232_DC"
                    n143 = property on="RS232 Config. System" class="Clust (strict)"("Visible"=w202) -> ()  [unwired: 2 in, 2 out]
                    n144 = property on="System ind." class="DigNum (strict)"("Visible"=w202) -> ()  [unwired: 2 in, 2 out]
                    n145 = property on="GPIB Configuration system" class="Clust (strict)"("Visible"=w201) -> ()  [unwired: 2 in, 2 out]
                    n146 = property on="TCP/IP Config. System" class="Clust (strict)"("Visible"=w201) -> ()  [unwired: 2 in, 2 out]
                  }
                  frame 6 {
                    w204 = FALSE ("Write Attribute")
                    # "USB_DC"
                    n147 = property on="TCP/IP Config. System" class="Clust (strict)"("Visible"=FALSE) -> ()  [unwired: 2 in, 2 out]
                    n148 = property on="GPIB Configuration system" class="Clust (strict)"("Visible"=w204) -> ()  [unwired: 2 in, 2 out]
                    n149 = property on="RS232 Config. System" class="Clust (strict)"("Visible"=w204) -> ()  [unwired: 2 in, 2 out]
                    n150 = property on="System ind." class="DigNum (strict)"("Visible"=w204) -> ()  [unwired: 2 in, 2 out]
                  }
                }
              }
            }
            n151 = property on="Send" class="Str"("Key Focus"=TRUE ("Write Attribute")) -> ()  [unwired: 2 in, 2 out]
          }
          frame True {
            n152 = Add(x=w213, y=1) -> (x+y=w209:i32)
            n153 = local read "Send"() -> (w221:string)
            n154 = String Length(string=w221) -> (length=w215:i32)
            n155 = Subtract(x=w215, y=w210) -> (x-y=w220:i32)
            n156 = String Subset(string=w221, offset (0)=w210, length (rest)=w220) -> (substring=w216:string)
            n157 = call "Analyse input string for terminal.vi"("Last string sent"=w222, "String new"=w216) -> ("String out"=w219:string, "Out not equal to in?"=w217:bool, "Attach term. char.?"=w205:bool)  [unwired: 15 out]
            n158 = case shown="True" w217 {
              tunnel: w219 -> [w234 w240]
              tunnel: [w231 w238] -> w214
              tunnel: w218 -> [w237 w241]
              tunnel: w216 -> [w236 _]
              frame True {
                n159 = Concatenate Strings(w237, w236, "  (Sent: " ("Substring"), w234, ")" ("Substring"), "\n") -> (w231:string)
                n160 = local write "Send"(w231) -> ()
              }
              frame False {
                n161 = Concatenate Strings(w241, w240, "\n") -> (w238:string)
                n162 = local write "Send"(w238) -> ()
              }
            }
            n163 = stacked-sequence {
              tunnel: [w229] -> w211
              tunnel: w214 -> [w230]
              frame #0 {
                n164 = String Length(string=w230) -> (length=w229:i32)
                n165 = property on="Send" class="Str"("Text.Selection:Start"=w229, "Text.Selection:End"=w229) -> ()  [unwired: 2 in, 2 out]
              }
            }
            n166 = stacked-sequence {
              tunnel: w211 -> [w226]
              tunnel: [w226] -> w208
              tunnel: w209 -> [w225]
              frame #0 {
                n167 = property on="Send" class="Str"("Text.Scroll Position"=w225) -> ()  [unwired: 2 in, 2 out]
              }
            }
            n168 = call "PI Send String.vi"("System no."=w224, "String to send"=w219, "Attach termination char.?"=w205) -> ("error out"=w206:errorcluster)  [unwired: 1 in, 15 out]
            "error out" <- w206
            n169 = stacked-sequence {
              tunnel: w208 -> [w227]
              tunnel: [w227] -> w207
              tunnel: w206 -> [_]
              frame #0 {
                n170 = property on="Send" class="Str"("Key Focus"=TRUE ("Write Attribute")) -> ()  [unwired: 2 in, 2 out]
              }
            }
            n171 = Unbundle By Name(w206) -> ("status"=w223:bool)
            n172 = local write "error"(w223) -> ()
          }
        }
        n173 = case shown="False" "Clear" {
          tunnel: [w144 ""] -> w110
          tunnel: w113 -> [w144 _]
          tunnel: [w143 0] -> w111
          tunnel: w112 -> [w143 _]
          frame False {
          }
          frame True {
            n174 = local write "Receive"("") -> ()
          }
        }
        n175 = case shown="0, Default" "View style" {
          tunnel: [u32 0 ("Write Attribute") u32 1 ("Write Attribute") u32 3 ("Write Attribute")] -> w125
          frame 0, Default {
          }
          frame 1 {
          }
          frame 2 {
          }
        }
        n176 = stacked-sequence {
          tunnel: w122 -> [_]
          tunnel: w121 -> [w162]
          tunnel: [w161] -> w120
          tunnel: [w160] -> w118
          tunnel: w110 -> [_]
          frame #0 {
            n177 = call "PI Receive String.vi"("System no."=w162, "Strip spaces?"=FALSE) -> ("String read"=w160:string, "bytes read"=w161:u16)  [unwired: 1 in, 15 out]
          }
        }
        n178 = property on="Receive" class="Str"("Display Style"=w125) -> ()  [unwired: 2 in, 2 out]
        n179 = Greater?(x=w120, y=u16 1) -> (0:w109:bool)
        n180 = case shown="True" w109 {
          tunnel: [w149 w155] -> w108
          tunnel: w118 -> [_ w157]
          tunnel: w110 -> [w149 w158]
          tunnel: [w148 w153] -> w106
          tunnel: w111 -> [w148 w154]
          frame False {
          }
          frame True {
            n181 = Concatenate Strings(w158, w157, "\n" ("string")) -> (w155:string)
            n182 = call "How often does string contain regular expression?.vi"("Regular expression"="\\n" ("regular expression"), "String"=w157) -> ("Number"=w152:i32)  [unwired: 17 out]
            n183 = Increment(x=w152) -> (x+1=w150:i32)
            n184 = local write "Receive"(w155) -> ()
            n185 = Add(x=w150, y=w154) -> (x+y=w153:i32)
          }
        }
        n186 = case shown="True" "Show help" {
          frame False {
          }
          frame True {
            n187 = property on="Send" class="Str"("Visible"=FALSE ("Write Attribute")) -> ()  [unwired: 2 in, 2 out]
            n188 = property on="String" class="Str"("Visible"=TRUE ("Write Attribute")) -> ()  [unwired: 2 in, 2 out]
            n189 = while {
              tunnel: [w138] -> w135
              stop <- w138 continue-if-true
              n190 = Not(x="Hide help") -> (.not. x?=w138:bool)
            }
            n191 = Not(x=w135) -> (.not. x?=w134:bool)
            n192 = property on="Send" class="Str"("Visible"=w134) -> ()  [unwired: 2 in, 2 out]
            n193 = property on="String" class="Str"("Visible"=w135) -> ()  [unwired: 2 in, 2 out]
          }
        }
        n194 = case shown="False" w109 {
          tunnel: w108 -> [w140 w142]
          tunnel: [w140 w142] -> w107
          tunnel: w106 -> [_ w141]
          frame False {
          }
          frame True {
            n195 = property on="Receive" class="Str"("Text.Scroll Position"=w141) -> ()  [unwired: 2 in, 2 out]
          }
        }
        n196 = local read "Exit"() -> (w104:bool)
        n197 = Not(x=w104) -> (.not. x?=w103:bool)
        n198 = Wait Until Next ms Multiple(millisecond multiple=u32 10) -> ()  [unwired: 1 out]
      }
      n199 = property on="Send" class="Str"("Key Focus"=TRUE ("Write Attribute")) -> ()  [unwired: 2 in, 2 out]
      n200 = local write "Exit"(w88) -> ()
    }
    frame #3 {
      n201 = case shown="True" "ERR? on exit?" {
        tunnel: w249 -> [_ w281]
        tunnel: w248 -> [_ w280]
        tunnel: w247 -> [_ w279]
        tunnel: w246 -> [_ w278]
        tunnel: w245 -> [_ w277]
        tunnel: ["" w254] -> w242
        frame False {
        }
        frame True {
          n202 = local read "System No."() -> (w273:i32)
          n203 = Add(x=w279, y=1) -> (x+y=w269:i32)
          n204 = local read "Send"() -> (w264:string)
          n205 = String Length(string=w264) -> (length=w261:i32)
          n206 = Subtract(x=w261, y=w281) -> (x-y=w263:i32)
          n207 = String Subset(string=w264, offset (0)=w281, length (rest)=w263) -> (substring=w262:string)
          n208 = call "Analyse input string for terminal.vi"("Last string sent"="ERR?", "String new"=w262) -> ("String out"=w276:string)  [unwired: 17 out]
          n209 = Concatenate Strings(w280, w262, "  (Sent: " ("Substring"), w276, ")" ("Substring"), "\n") -> (w275:string)
          n210 = stacked-sequence {
            tunnel: [w287] -> w259
            tunnel: w275 -> [w288]
            frame #0 {
              n211 = String Length(string=w288) -> (length=w287:i32)
              n212 = property on="Send" class="Str"("Text.Selection:Start"=w287, "Text.Selection:End"=w287) -> ()  [unwired: 2 in, 2 out]
            }
          }
          n213 = stacked-sequence {
            tunnel: w259 -> [w284]
            tunnel: [w284] -> w258
            tunnel: w269 -> [w283]
            frame #0 {
              n214 = property on="Send" class="Str"("Text.Scroll Position"=w283) -> ()  [unwired: 2 in, 2 out]
            }
          }
          n215 = stacked-sequence {
            tunnel: w258 -> [w285]
            tunnel: [w285] -> w274
            frame #0 {
              n216 = property on="Send" class="Str"("Key Focus"=TRUE ("Write Attribute")) -> ()  [unwired: 2 in, 2 out]
            }
          }
          n217 = stacked-sequence {
            tunnel: w274 -> [_]
            tunnel: w273 -> [w303]
            tunnel: [w302] -> w272
            tunnel: [w301] -> w270
            tunnel: w278 -> [_]
            frame #0 {
              n218 = call "PI Receive String.vi"("System no."=w303) -> ("String read"=w301:string, "bytes read"=w302:u16)  [unwired: 2 in, 15 out]
            }
          }
          n219 = Greater?(x=w272, y=u16 1) -> (0:w268:bool)
          n220 = case shown="True" w268 {
            tunnel: [w293 w297] -> w267
            tunnel: w270 -> [_ w299]
            tunnel: w278 -> [w293 w300]
            tunnel: [w292 w294] -> w266
            tunnel: w277 -> [w292 w295]
            frame False {
            }
            frame True {
              n221 = Concatenate Strings(w300, w299) -> (w297:string)
              n222 = call "How often does string contain regular expression?.vi"("Regular expression"="\\n" ("regular expression"), "String"=w299) -> ("Number"=w296:i32)  [unwired: 17 out]
              n223 = local write "Receive"(w297) -> ()
              n224 = Add(x=w296, y=w295) -> (x+y=w294:i32)
            }
          }
          n225 = local write "Send"(w275) -> ()
          n226 = call "PI Send String.vi"("System no."=w273, "String to send"=w276, "Attach termination char.?"=TRUE ("Attach Linefeed?")) -> ()  [unwired: 1 in, 16 out]
          n227 = case shown="True" w268 {
            tunnel: w267 -> [w289 w291]
            tunnel: [w289 w291] -> w254
            tunnel: w266 -> [_ w290]
            frame False {
            }
            frame True {
              n228 = property on="Receive" class="Str"("Text.Scroll Position"=w290) -> ()  [unwired: 2 in, 2 out]
            }
          }
        }
      }
      n229 = for {
        N: w243 -> [_]
        tunnel: w242 -> [_]
        i -> [w252]
        n230 = Increment(x=w252) -> (x+1=w251:i32)
        n231 = call "Close connection if open.vi"("System no."=w251, "Close DaisyChain"=TRUE) -> ()  [unwired: 1 in, 17 out]
      }
    }
  }
